vi "Experiment 18.vi"() -> ()   [LabVIEW 2026]
doc: "Experiment 18\nThis experiment is like Experiment 12 but contains only 8 parallel loops (instead of 10 as in Exp 12)."
uses:
  <vilib>/AdvancedString/1D String Array to Delimited String (string).vi
  <vilib>/Analysis/baseanly.llb/Mean (DBL).vi
  <vilib>/Analysis/NI_AALBase.lvlib
panel:
  out "No. Of Iterations As Block Of Text (easy to copy into Excel)":string
  out "No. Of Iterations Executed - Loop 8":i32
  out "Output - Loop 8":dbl[](array[numeric]) format="%.3f"
  out "No. Of Iterations Executed - Loop 7":i32
  out "Output - Loop 7":dbl[](array[numeric]) format="%.3f"
  out "No. Of Iterations Executed - Loop 6":i32
  out "Output - Loop 6":dbl[](array[numeric]) format="%.3f"
  out "No. Of Iterations Executed - Loop 5":i32
  out "Output - Loop 5":dbl[](array[numeric]) format="%.3f"
  out "No. Of Iterations Executed - Loop 4":i32
  out "Output - Loop 4":dbl[](array[numeric]) format="%.3f"
  out "No. Of Iterations Executed - Loop 3":i32
  out "Output - Loop 3":dbl[](array[numeric]) format="%.3f"
  out "Avg. No. Of Iterations Executed - All Loops":dbl format="%.1f"
  out "No. Of Iterations Executed - Loop 2":i32
  out "Output - Loop 2":dbl[](array[numeric]) format="%.3f"
  out "No. Of Iterations Executed - Loop 1":i32
  out "Output - Loop 1":dbl[](array[numeric]) format="%.3f"
  out "Stop VI?":bool
  # "Experiment 18"
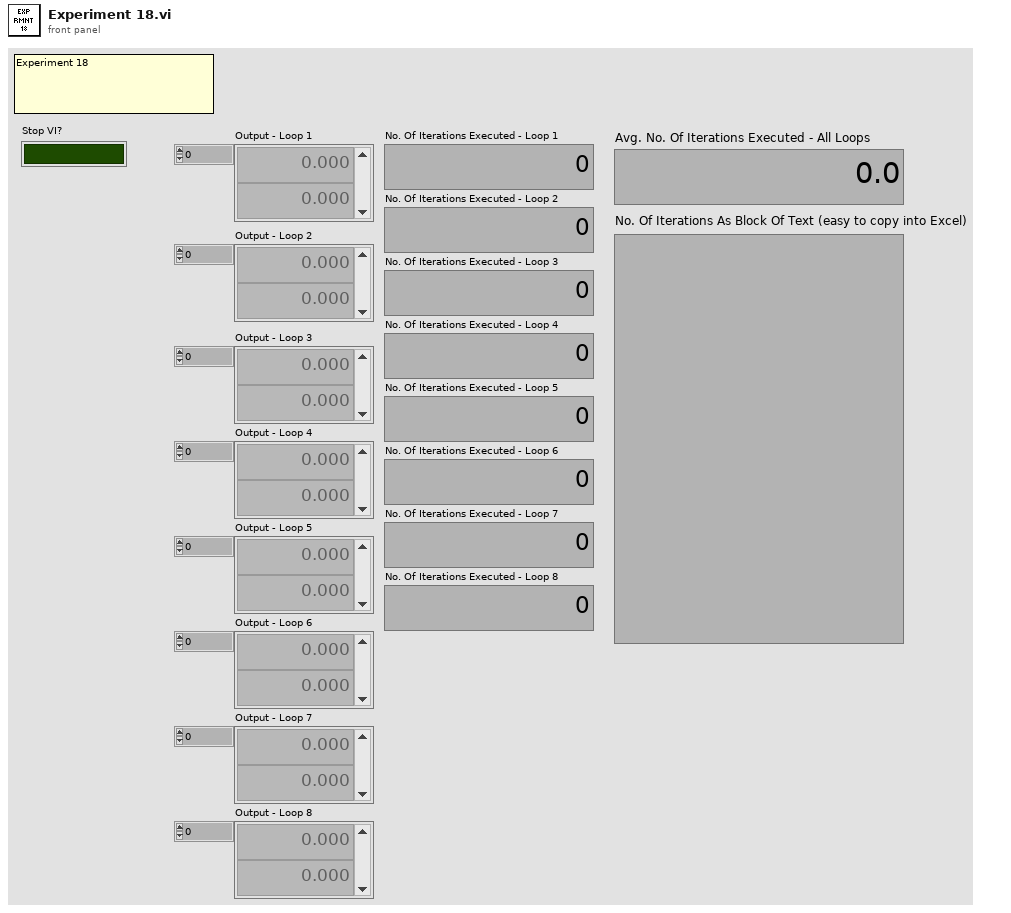
[diagram p1: front panel]
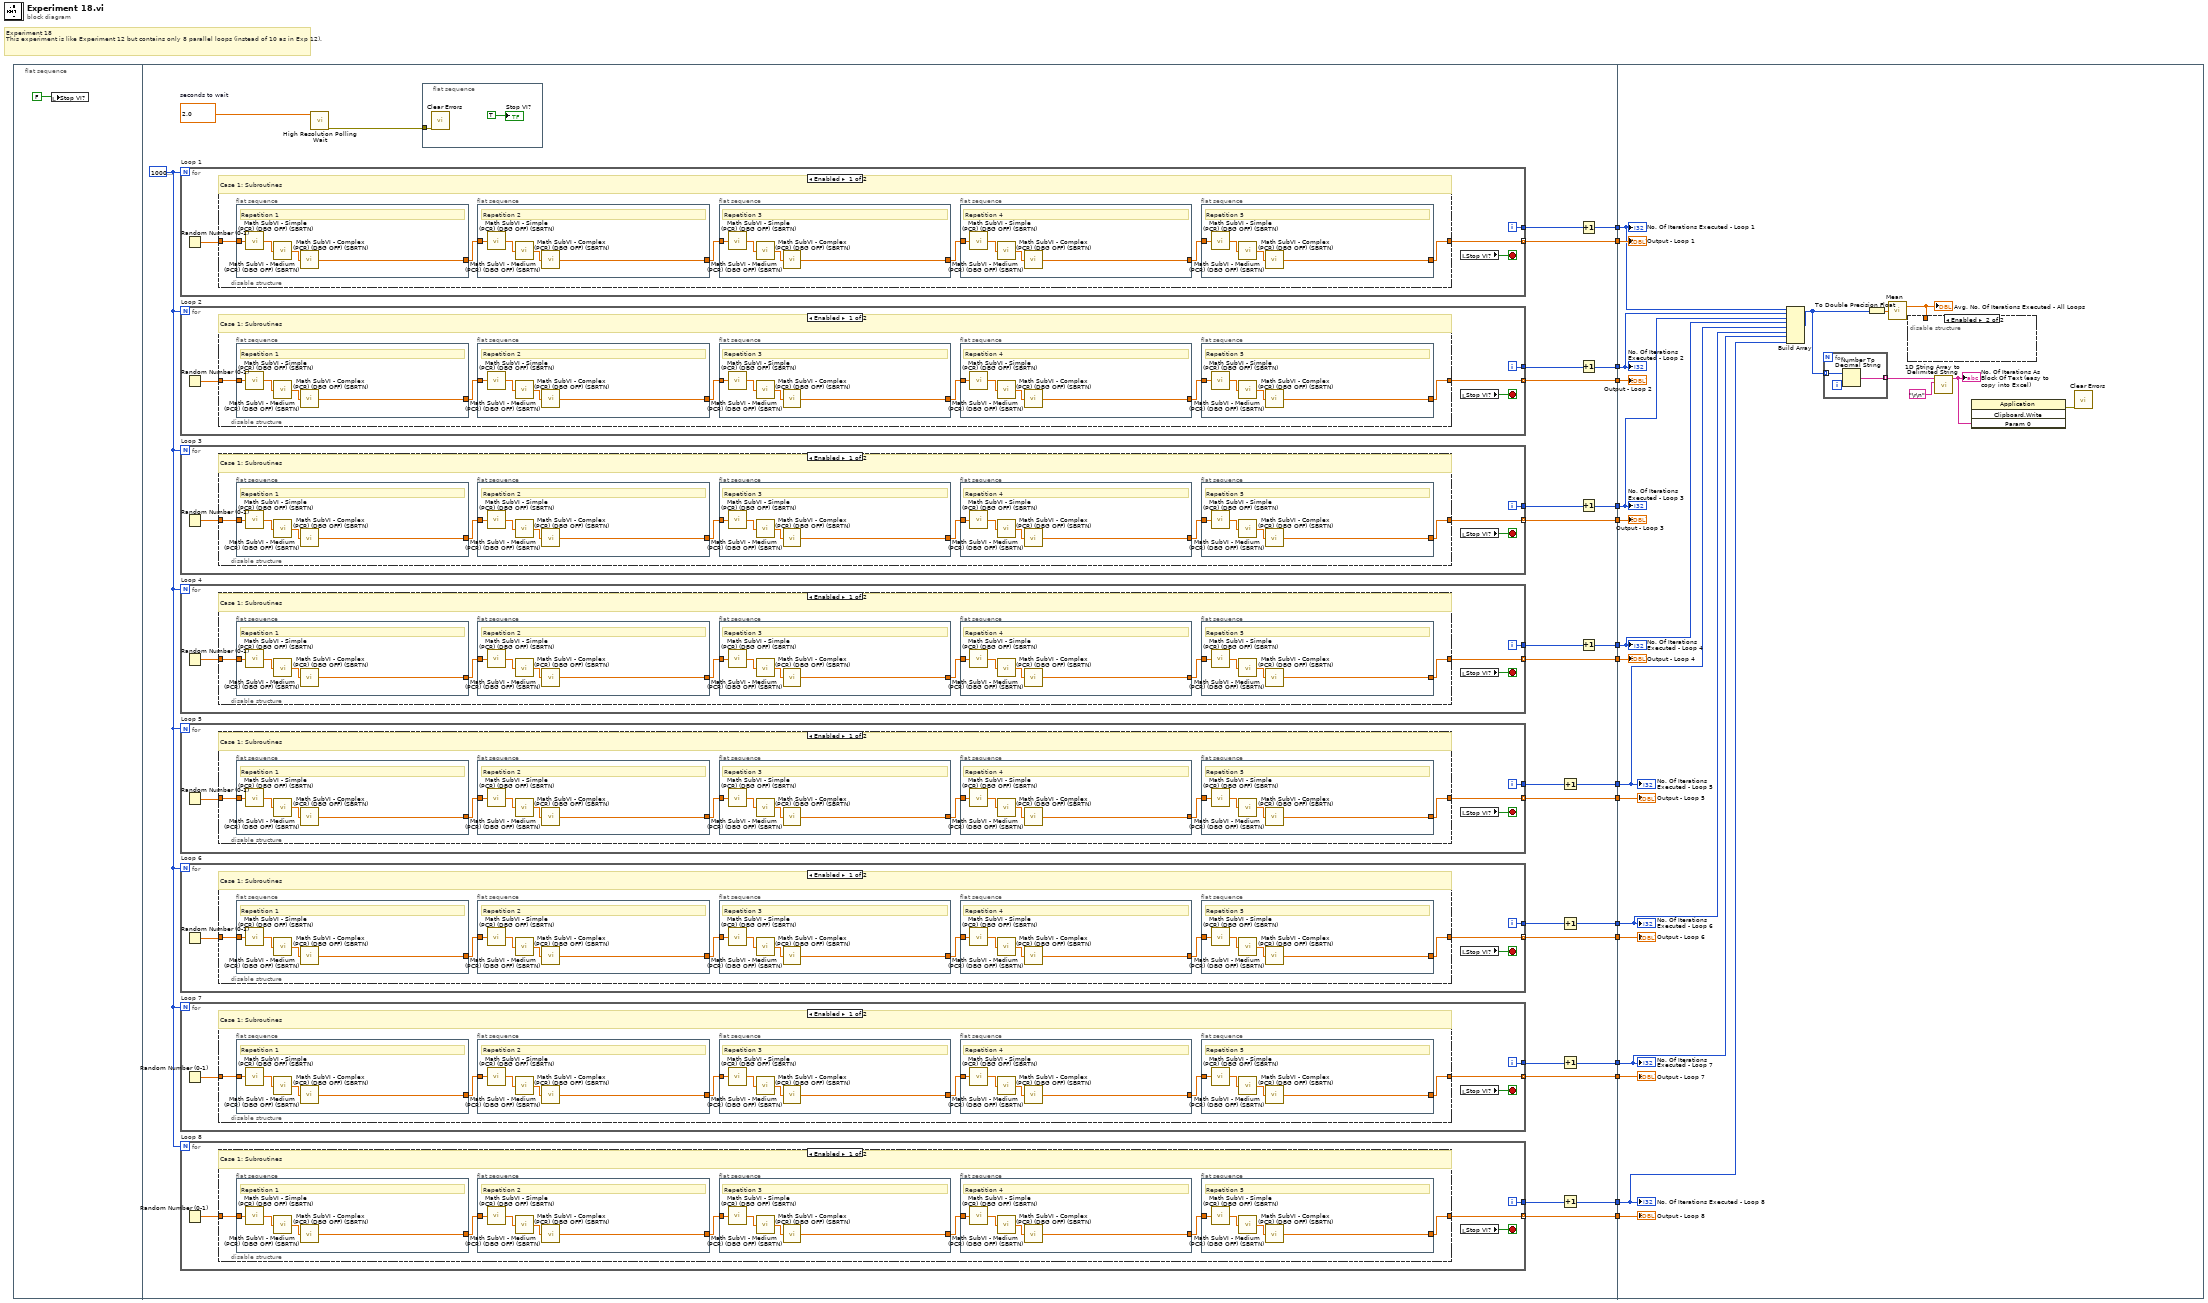
[diagram p0: block diagram]
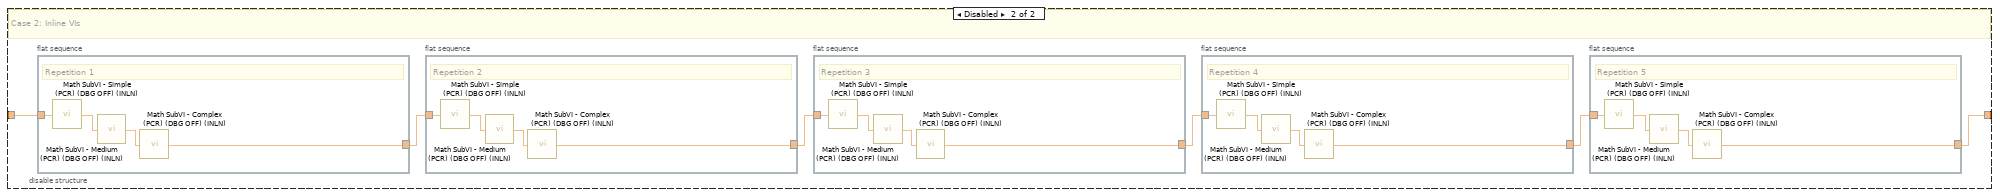
[diagram p2: hidden frame]
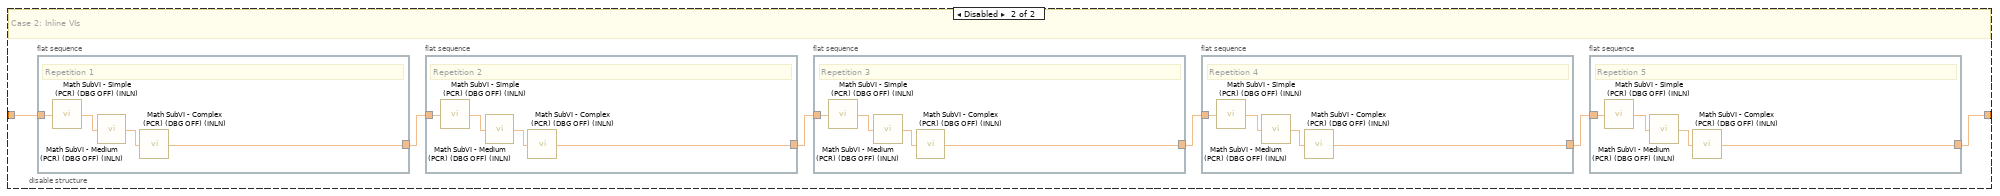
[diagram p3: hidden frame]
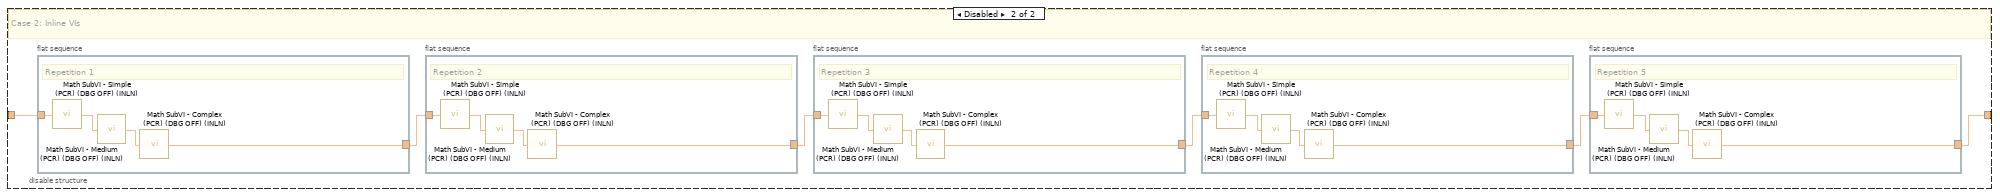
[diagram p4: hidden frame]
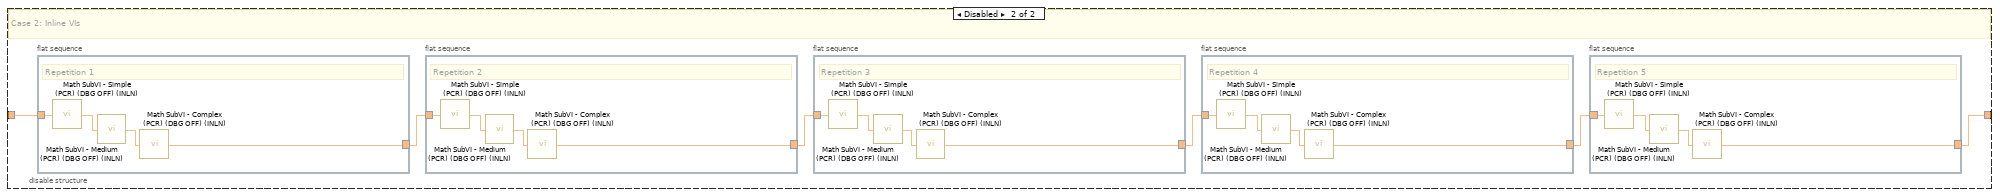
[diagram p5: hidden frame]
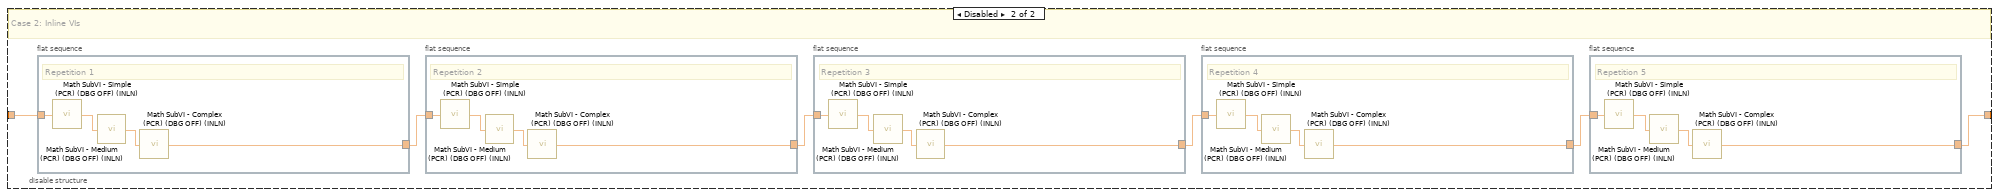
[diagram p6: hidden frame]
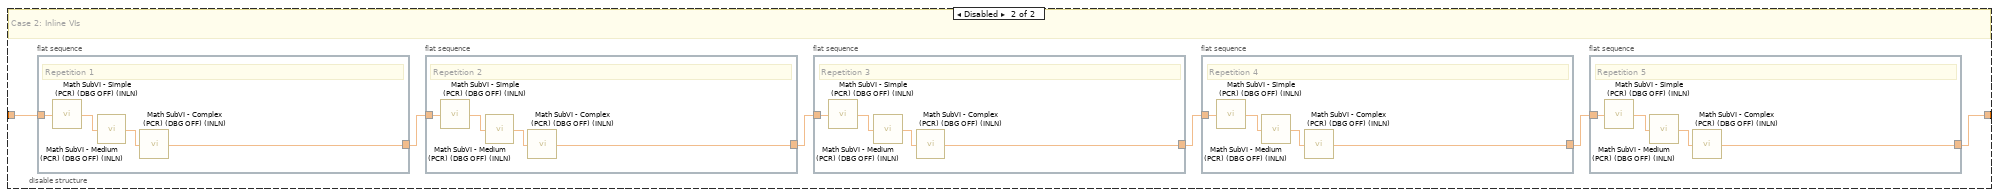
[diagram p7: hidden frame]
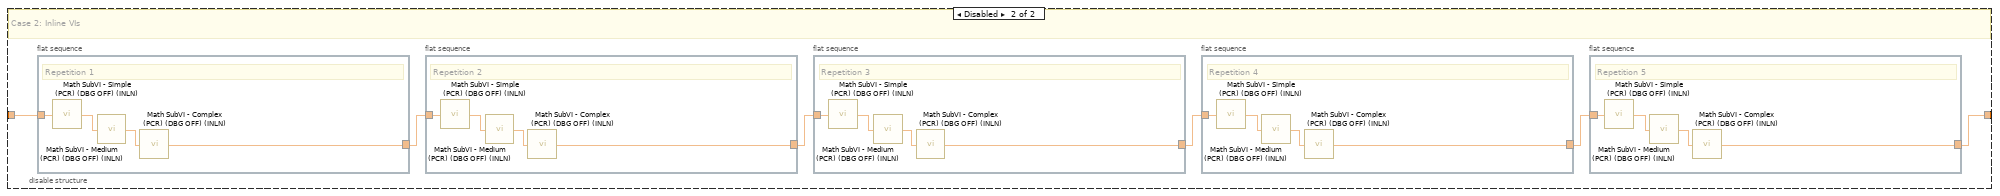
[diagram p8: hidden frame]
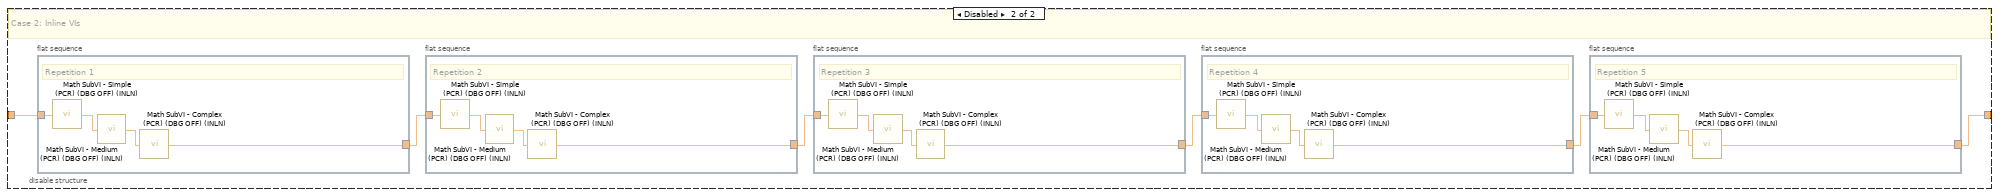
[diagram p9: hidden frame]
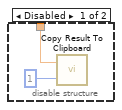
[diagram p10: hidden frame]
diagram:
  # "Experiment 18\nThis experiment is like Experiment 12 but contains only 8 parallel loops (instead of 10 as in Exp 12)."
  n1 = flat-sequence {
    tunnel: [w42] -> w16
    tunnel: [w40] -> w15
    tunnel: [w39] -> w14
    tunnel: [w32] -> w13
    tunnel: [w38] -> w12
    tunnel: [w30] -> w11
    tunnel: [w28] -> w10
    tunnel: [w37] -> w9
    tunnel: [w26] -> w8
    tunnel: [w36] -> w7
    tunnel: [w24] -> w6
    tunnel: [w33] -> w5
    tunnel: [w22] -> w4
    tunnel: [w34] -> w3
    tunnel: [w19] -> w2
    tunnel: [w35] -> w1
    tunnel: w16 -> [w517]
    tunnel: w15 -> [w515]
    tunnel: w14 -> [w514]
    tunnel: w13 -> [w516]
    tunnel: w12 -> [w510]
    tunnel: w11 -> [w512]
    tunnel: w10 -> [w511]
    tunnel: w9 -> [w509]
    tunnel: w8 -> [w507]
    tunnel: w7 -> [w503]
    tunnel: w6 -> [w506]
    tunnel: w5 -> [w502]
    tunnel: w4 -> [w505]
    tunnel: w3 -> [w501]
    tunnel: w2 -> [w504]
    tunnel: w1 -> [w500]
    frame #0 {
      n2 = local write "Stop VI?"(FALSE) -> ()
    }
    frame #1 {
      w18 = 10000000
      w44 = 2.0  # seconds to wait
      n3 = for "Loop 1" {
        N: w18 -> [_]
        tunnel: [w440] -> w42 mode=indexing
        tunnel: [w441] -> w41
        i -> [w441]
        stop <- w442 stop-if-true
        n4 = Random Number (0-1)() -> (number: 0 to 1=w439:dbl)
        n5 = disable-structure shown="Enabled" {
          disable-tunnel: w439 -> [w448 w474]
          disable-tunnel: [w447 w469] -> w440
          frame Enabled {
            # "Case 1: Subroutines"
            n6 = flat-sequence {
              tunnel: w448 -> [w468]
              tunnel: [w465] -> w443
              frame #0 {
                # "Repetition 1"
                n7 = call "Math SubVI - Simple (PCR) (DBG OFF) (SBRTN).vi"("Input"=w468) -> ("Output"=w466:dbl)
                n8 = call "Math SubVI - Medium (PCR) (DBG OFF) (SBRTN).vi"("Input"=w466) -> ("Output"=w467:dbl)
                n9 = call "Math SubVI - Complex (PCR) (DBG OFF) (SBRTN).vi"("Input"=w467) -> ("Output"=w465:dbl)
              }
            }
            n10 = flat-sequence {
              tunnel: w443 -> [w464]
              tunnel: [w461] -> w446
              frame #0 {
                # "Repetition 2"
                n11 = call "Math SubVI - Simple (PCR) (DBG OFF) (SBRTN).vi"("Input"=w464) -> ("Output"=w462:dbl)
                n12 = call "Math SubVI - Medium (PCR) (DBG OFF) (SBRTN).vi"("Input"=w462) -> ("Output"=w463:dbl)
                n13 = call "Math SubVI - Complex (PCR) (DBG OFF) (SBRTN).vi"("Input"=w463) -> ("Output"=w461:dbl)
              }
            }
            n14 = flat-sequence {
              tunnel: w446 -> [w460]
              tunnel: [w457] -> w445
              frame #0 {
                # "Repetition 3"
                n15 = call "Math SubVI - Simple (PCR) (DBG OFF) (SBRTN).vi"("Input"=w460) -> ("Output"=w458:dbl)
                n16 = call "Math SubVI - Medium (PCR) (DBG OFF) (SBRTN).vi"("Input"=w458) -> ("Output"=w459:dbl)
                n17 = call "Math SubVI - Complex (PCR) (DBG OFF) (SBRTN).vi"("Input"=w459) -> ("Output"=w457:dbl)
              }
            }
            n18 = flat-sequence {
              tunnel: w445 -> [w456]
              tunnel: [w453] -> w444
              frame #0 {
                # "Repetition 4"
                n19 = call "Math SubVI - Simple (PCR) (DBG OFF) (SBRTN).vi"("Input"=w456) -> ("Output"=w454:dbl)
                n20 = call "Math SubVI - Medium (PCR) (DBG OFF) (SBRTN).vi"("Input"=w454) -> ("Output"=w455:dbl)
                n21 = call "Math SubVI - Complex (PCR) (DBG OFF) (SBRTN).vi"("Input"=w455) -> ("Output"=w453:dbl)
              }
            }
            n22 = flat-sequence {
              tunnel: w444 -> [w452]
              tunnel: [w449] -> w447
              frame #0 {
                # "Repetition 5"
                n23 = call "Math SubVI - Simple (PCR) (DBG OFF) (SBRTN).vi"("Input"=w452) -> ("Output"=w450:dbl)
                n24 = call "Math SubVI - Medium (PCR) (DBG OFF) (SBRTN).vi"("Input"=w450) -> ("Output"=w451:dbl)
                n25 = call "Math SubVI - Complex (PCR) (DBG OFF) (SBRTN).vi"("Input"=w451) -> ("Output"=w449:dbl)
              }
            }
          }
          frame Disabled {
            # "Case 2: Inline VIs"
            n26 = flat-sequence {
              tunnel: w474 -> [w494]
              tunnel: [w491] -> w473
              frame #0 {
                # "Repetition 1"
                n27 = call "Math SubVI - Simple (PCR) (DBG OFF) (INLN).vi"("Input"=w494) -> ("Output"=w492:dbl)
                n28 = call "Math SubVI - Medium (PCR) (DBG OFF) (INLN).vi"("Input"=w492) -> ("Output"=w493:dbl)
                n29 = call "Math SubVI - Complex (PCR) (DBG OFF) (INLN).vi"("Input"=w493) -> ("Output"=w491:dbl)
              }
            }
            n30 = flat-sequence {
              tunnel: w473 -> [w490]
              tunnel: [w487] -> w472
              frame #0 {
                # "Repetition 2"
                n31 = call "Math SubVI - Simple (PCR) (DBG OFF) (INLN).vi"("Input"=w490) -> ("Output"=w488:dbl)
                n32 = call "Math SubVI - Medium (PCR) (DBG OFF) (INLN).vi"("Input"=w488) -> ("Output"=w489:dbl)
                n33 = call "Math SubVI - Complex (PCR) (DBG OFF) (INLN).vi"("Input"=w489) -> ("Output"=w487:dbl)
              }
            }
            n34 = flat-sequence {
              tunnel: w472 -> [w486]
              tunnel: [w483] -> w471
              frame #0 {
                # "Repetition 3"
                n35 = call "Math SubVI - Simple (PCR) (DBG OFF) (INLN).vi"("Input"=w486) -> ("Output"=w484:dbl)
                n36 = call "Math SubVI - Medium (PCR) (DBG OFF) (INLN).vi"("Input"=w484) -> ("Output"=w485:dbl)
                n37 = call "Math SubVI - Complex (PCR) (DBG OFF) (INLN).vi"("Input"=w485) -> ("Output"=w483:dbl)
              }
            }
            n38 = flat-sequence {
              tunnel: w471 -> [w482]
              tunnel: [w479] -> w470
              frame #0 {
                # "Repetition 4"
                n39 = call "Math SubVI - Simple (PCR) (DBG OFF) (INLN).vi"("Input"=w482) -> ("Output"=w480:dbl)
                n40 = call "Math SubVI - Medium (PCR) (DBG OFF) (INLN).vi"("Input"=w480) -> ("Output"=w481:dbl)
                n41 = call "Math SubVI - Complex (PCR) (DBG OFF) (INLN).vi"("Input"=w481) -> ("Output"=w479:dbl)
              }
            }
            n42 = flat-sequence {
              tunnel: w470 -> [w478]
              tunnel: [w475] -> w469
              frame #0 {
                # "Repetition 5"
                n43 = call "Math SubVI - Simple (PCR) (DBG OFF) (INLN).vi"("Input"=w478) -> ("Output"=w476:dbl)
                n44 = call "Math SubVI - Medium (PCR) (DBG OFF) (INLN).vi"("Input"=w476) -> ("Output"=w477:dbl)
                n45 = call "Math SubVI - Complex (PCR) (DBG OFF) (INLN).vi"("Input"=w477) -> ("Output"=w475:dbl)
              }
            }
          }
        }
        n46 = local read "Stop VI?"() -> (w442:bool)
      }
      n47 = for "Loop 2" {
        N: w18 -> [_]
        tunnel: [w384] -> w32 mode=indexing
        tunnel: [w385] -> w31
        i -> [w385]
        stop <- w386 stop-if-true
        n48 = Random Number (0-1)() -> (number: 0 to 1=w383:dbl)
        n49 = disable-structure shown="Enabled" {
          disable-tunnel: w383 -> [w392 w418]
          disable-tunnel: [w391 w413] -> w384
          frame Enabled {
            # "Case 1: Subroutines"
            n50 = flat-sequence {
              tunnel: w392 -> [w412]
              tunnel: [w409] -> w387
              frame #0 {
                # "Repetition 1"
                n51 = call "Math SubVI - Simple (PCR) (DBG OFF) (SBRTN).vi"("Input"=w412) -> ("Output"=w410:dbl)
                n52 = call "Math SubVI - Medium (PCR) (DBG OFF) (SBRTN).vi"("Input"=w410) -> ("Output"=w411:dbl)
                n53 = call "Math SubVI - Complex (PCR) (DBG OFF) (SBRTN).vi"("Input"=w411) -> ("Output"=w409:dbl)
              }
            }
            n54 = flat-sequence {
              tunnel: w387 -> [w408]
              tunnel: [w405] -> w390
              frame #0 {
                # "Repetition 2"
                n55 = call "Math SubVI - Simple (PCR) (DBG OFF) (SBRTN).vi"("Input"=w408) -> ("Output"=w406:dbl)
                n56 = call "Math SubVI - Medium (PCR) (DBG OFF) (SBRTN).vi"("Input"=w406) -> ("Output"=w407:dbl)
                n57 = call "Math SubVI - Complex (PCR) (DBG OFF) (SBRTN).vi"("Input"=w407) -> ("Output"=w405:dbl)
              }
            }
            n58 = flat-sequence {
              tunnel: w390 -> [w404]
              tunnel: [w401] -> w389
              frame #0 {
                # "Repetition 3"
                n59 = call "Math SubVI - Simple (PCR) (DBG OFF) (SBRTN).vi"("Input"=w404) -> ("Output"=w402:dbl)
                n60 = call "Math SubVI - Medium (PCR) (DBG OFF) (SBRTN).vi"("Input"=w402) -> ("Output"=w403:dbl)
                n61 = call "Math SubVI - Complex (PCR) (DBG OFF) (SBRTN).vi"("Input"=w403) -> ("Output"=w401:dbl)
              }
            }
            n62 = flat-sequence {
              tunnel: w389 -> [w400]
              tunnel: [w397] -> w388
              frame #0 {
                # "Repetition 4"
                n63 = call "Math SubVI - Simple (PCR) (DBG OFF) (SBRTN).vi"("Input"=w400) -> ("Output"=w398:dbl)
                n64 = call "Math SubVI - Medium (PCR) (DBG OFF) (SBRTN).vi"("Input"=w398) -> ("Output"=w399:dbl)
                n65 = call "Math SubVI - Complex (PCR) (DBG OFF) (SBRTN).vi"("Input"=w399) -> ("Output"=w397:dbl)
              }
            }
            n66 = flat-sequence {
              tunnel: w388 -> [w396]
              tunnel: [w393] -> w391
              frame #0 {
                # "Repetition 5"
                n67 = call "Math SubVI - Simple (PCR) (DBG OFF) (SBRTN).vi"("Input"=w396) -> ("Output"=w394:dbl)
                n68 = call "Math SubVI - Medium (PCR) (DBG OFF) (SBRTN).vi"("Input"=w394) -> ("Output"=w395:dbl)
                n69 = call "Math SubVI - Complex (PCR) (DBG OFF) (SBRTN).vi"("Input"=w395) -> ("Output"=w393:dbl)
              }
            }
          }
          frame Disabled {
            # "Case 2: Inline VIs"
            n70 = flat-sequence {
              tunnel: w418 -> [w438]
              tunnel: [w435] -> w417
              frame #0 {
                # "Repetition 1"
                n71 = call "Math SubVI - Simple (PCR) (DBG OFF) (INLN).vi"("Input"=w438) -> ("Output"=w436:dbl)
                n72 = call "Math SubVI - Medium (PCR) (DBG OFF) (INLN).vi"("Input"=w436) -> ("Output"=w437:dbl)
                n73 = call "Math SubVI - Complex (PCR) (DBG OFF) (INLN).vi"("Input"=w437) -> ("Output"=w435:dbl)
              }
            }
            n74 = flat-sequence {
              tunnel: w417 -> [w434]
              tunnel: [w431] -> w416
              frame #0 {
                # "Repetition 2"
                n75 = call "Math SubVI - Simple (PCR) (DBG OFF) (INLN).vi"("Input"=w434) -> ("Output"=w432:dbl)
                n76 = call "Math SubVI - Medium (PCR) (DBG OFF) (INLN).vi"("Input"=w432) -> ("Output"=w433:dbl)
                n77 = call "Math SubVI - Complex (PCR) (DBG OFF) (INLN).vi"("Input"=w433) -> ("Output"=w431:dbl)
              }
            }
            n78 = flat-sequence {
              tunnel: w416 -> [w430]
              tunnel: [w427] -> w415
              frame #0 {
                # "Repetition 3"
                n79 = call "Math SubVI - Simple (PCR) (DBG OFF) (INLN).vi"("Input"=w430) -> ("Output"=w428:dbl)
                n80 = call "Math SubVI - Medium (PCR) (DBG OFF) (INLN).vi"("Input"=w428) -> ("Output"=w429:dbl)
                n81 = call "Math SubVI - Complex (PCR) (DBG OFF) (INLN).vi"("Input"=w429) -> ("Output"=w427:dbl)
              }
            }
            n82 = flat-sequence {
              tunnel: w415 -> [w426]
              tunnel: [w423] -> w414
              frame #0 {
                # "Repetition 4"
                n83 = call "Math SubVI - Simple (PCR) (DBG OFF) (INLN).vi"("Input"=w426) -> ("Output"=w424:dbl)
                n84 = call "Math SubVI - Medium (PCR) (DBG OFF) (INLN).vi"("Input"=w424) -> ("Output"=w425:dbl)
                n85 = call "Math SubVI - Complex (PCR) (DBG OFF) (INLN).vi"("Input"=w425) -> ("Output"=w423:dbl)
              }
            }
            n86 = flat-sequence {
              tunnel: w414 -> [w422]
              tunnel: [w419] -> w413
              frame #0 {
                # "Repetition 5"
                n87 = call "Math SubVI - Simple (PCR) (DBG OFF) (INLN).vi"("Input"=w422) -> ("Output"=w420:dbl)
                n88 = call "Math SubVI - Medium (PCR) (DBG OFF) (INLN).vi"("Input"=w420) -> ("Output"=w421:dbl)
                n89 = call "Math SubVI - Complex (PCR) (DBG OFF) (INLN).vi"("Input"=w421) -> ("Output"=w419:dbl)
              }
            }
          }
        }
        n90 = local read "Stop VI?"() -> (w386:bool)
      }
      n91 = for "Loop 3" {
        N: w18 -> [_]
        tunnel: [w328] -> w30 mode=indexing
        tunnel: [w329] -> w29
        i -> [w329]
        stop <- w330 stop-if-true
        n92 = Random Number (0-1)() -> (number: 0 to 1=w327:dbl)
        n93 = disable-structure shown="Enabled" {
          disable-tunnel: w327 -> [w336 w362]
          disable-tunnel: [w335 w357] -> w328
          frame Enabled {
            # "Case 1: Subroutines"
            n94 = flat-sequence {
              tunnel: w336 -> [w356]
              tunnel: [w353] -> w331
              frame #0 {
                # "Repetition 1"
                n95 = call "Math SubVI - Simple (PCR) (DBG OFF) (SBRTN).vi"("Input"=w356) -> ("Output"=w354:dbl)
                n96 = call "Math SubVI - Medium (PCR) (DBG OFF) (SBRTN).vi"("Input"=w354) -> ("Output"=w355:dbl)
                n97 = call "Math SubVI - Complex (PCR) (DBG OFF) (SBRTN).vi"("Input"=w355) -> ("Output"=w353:dbl)
              }
            }
            n98 = flat-sequence {
              tunnel: w331 -> [w352]
              tunnel: [w349] -> w334
              frame #0 {
                # "Repetition 2"
                n99 = call "Math SubVI - Simple (PCR) (DBG OFF) (SBRTN).vi"("Input"=w352) -> ("Output"=w350:dbl)
                n100 = call "Math SubVI - Medium (PCR) (DBG OFF) (SBRTN).vi"("Input"=w350) -> ("Output"=w351:dbl)
                n101 = call "Math SubVI - Complex (PCR) (DBG OFF) (SBRTN).vi"("Input"=w351) -> ("Output"=w349:dbl)
              }
            }
            n102 = flat-sequence {
              tunnel: w334 -> [w348]
              tunnel: [w345] -> w333
              frame #0 {
                # "Repetition 3"
                n103 = call "Math SubVI - Simple (PCR) (DBG OFF) (SBRTN).vi"("Input"=w348) -> ("Output"=w346:dbl)
                n104 = call "Math SubVI - Medium (PCR) (DBG OFF) (SBRTN).vi"("Input"=w346) -> ("Output"=w347:dbl)
                n105 = call "Math SubVI - Complex (PCR) (DBG OFF) (SBRTN).vi"("Input"=w347) -> ("Output"=w345:dbl)
              }
            }
            n106 = flat-sequence {
              tunnel: w333 -> [w344]
              tunnel: [w341] -> w332
              frame #0 {
                # "Repetition 4"
                n107 = call "Math SubVI - Simple (PCR) (DBG OFF) (SBRTN).vi"("Input"=w344) -> ("Output"=w342:dbl)
                n108 = call "Math SubVI - Medium (PCR) (DBG OFF) (SBRTN).vi"("Input"=w342) -> ("Output"=w343:dbl)
                n109 = call "Math SubVI - Complex (PCR) (DBG OFF) (SBRTN).vi"("Input"=w343) -> ("Output"=w341:dbl)
              }
            }
            n110 = flat-sequence {
              tunnel: w332 -> [w340]
              tunnel: [w337] -> w335
              frame #0 {
                # "Repetition 5"
                n111 = call "Math SubVI - Simple (PCR) (DBG OFF) (SBRTN).vi"("Input"=w340) -> ("Output"=w338:dbl)
                n112 = call "Math SubVI - Medium (PCR) (DBG OFF) (SBRTN).vi"("Input"=w338) -> ("Output"=w339:dbl)
                n113 = call "Math SubVI - Complex (PCR) (DBG OFF) (SBRTN).vi"("Input"=w339) -> ("Output"=w337:dbl)
              }
            }
          }
          frame Disabled {
            # "Case 2: Inline VIs"
            n114 = flat-sequence {
              tunnel: w362 -> [w382]
              tunnel: [w379] -> w361
              frame #0 {
                # "Repetition 1"
                n115 = call "Math SubVI - Simple (PCR) (DBG OFF) (INLN).vi"("Input"=w382) -> ("Output"=w380:dbl)
                n116 = call "Math SubVI - Medium (PCR) (DBG OFF) (INLN).vi"("Input"=w380) -> ("Output"=w381:dbl)
                n117 = call "Math SubVI - Complex (PCR) (DBG OFF) (INLN).vi"("Input"=w381) -> ("Output"=w379:dbl)
              }
            }
            n118 = flat-sequence {
              tunnel: w361 -> [w378]
              tunnel: [w375] -> w360
              frame #0 {
                # "Repetition 2"
                n119 = call "Math SubVI - Simple (PCR) (DBG OFF) (INLN).vi"("Input"=w378) -> ("Output"=w376:dbl)
                n120 = call "Math SubVI - Medium (PCR) (DBG OFF) (INLN).vi"("Input"=w376) -> ("Output"=w377:dbl)
                n121 = call "Math SubVI - Complex (PCR) (DBG OFF) (INLN).vi"("Input"=w377) -> ("Output"=w375:dbl)
              }
            }
            n122 = flat-sequence {
              tunnel: w360 -> [w374]
              tunnel: [w371] -> w359
              frame #0 {
                # "Repetition 3"
                n123 = call "Math SubVI - Simple (PCR) (DBG OFF) (INLN).vi"("Input"=w374) -> ("Output"=w372:dbl)
                n124 = call "Math SubVI - Medium (PCR) (DBG OFF) (INLN).vi"("Input"=w372) -> ("Output"=w373:dbl)
                n125 = call "Math SubVI - Complex (PCR) (DBG OFF) (INLN).vi"("Input"=w373) -> ("Output"=w371:dbl)
              }
            }
            n126 = flat-sequence {
              tunnel: w359 -> [w370]
              tunnel: [w367] -> w358
              frame #0 {
                # "Repetition 4"
                n127 = call "Math SubVI - Simple (PCR) (DBG OFF) (INLN).vi"("Input"=w370) -> ("Output"=w368:dbl)
                n128 = call "Math SubVI - Medium (PCR) (DBG OFF) (INLN).vi"("Input"=w368) -> ("Output"=w369:dbl)
                n129 = call "Math SubVI - Complex (PCR) (DBG OFF) (INLN).vi"("Input"=w369) -> ("Output"=w367:dbl)
              }
            }
            n130 = flat-sequence {
              tunnel: w358 -> [w366]
              tunnel: [w363] -> w357
              frame #0 {
                # "Repetition 5"
                n131 = call "Math SubVI - Simple (PCR) (DBG OFF) (INLN).vi"("Input"=w366) -> ("Output"=w364:dbl)
                n132 = call "Math SubVI - Medium (PCR) (DBG OFF) (INLN).vi"("Input"=w364) -> ("Output"=w365:dbl)
                n133 = call "Math SubVI - Complex (PCR) (DBG OFF) (INLN).vi"("Input"=w365) -> ("Output"=w363:dbl)
              }
            }
          }
        }
        n134 = local read "Stop VI?"() -> (w330:bool)
      }
      n135 = for "Loop 4" {
        N: w18 -> [_]
        tunnel: [w272] -> w28 mode=indexing
        tunnel: [w273] -> w27
        i -> [w273]
        stop <- w274 stop-if-true
        n136 = Random Number (0-1)() -> (number: 0 to 1=w271:dbl)
        n137 = disable-structure shown="Enabled" {
          disable-tunnel: w271 -> [w280 w306]
          disable-tunnel: [w279 w301] -> w272
          frame Enabled {
            # "Case 1: Subroutines"
            n138 = flat-sequence {
              tunnel: w280 -> [w300]
              tunnel: [w297] -> w275
              frame #0 {
                # "Repetition 1"
                n139 = call "Math SubVI - Simple (PCR) (DBG OFF) (SBRTN).vi"("Input"=w300) -> ("Output"=w298:dbl)
                n140 = call "Math SubVI - Medium (PCR) (DBG OFF) (SBRTN).vi"("Input"=w298) -> ("Output"=w299:dbl)
                n141 = call "Math SubVI - Complex (PCR) (DBG OFF) (SBRTN).vi"("Input"=w299) -> ("Output"=w297:dbl)
              }
            }
            n142 = flat-sequence {
              tunnel: w275 -> [w296]
              tunnel: [w293] -> w278
              frame #0 {
                # "Repetition 2"
                n143 = call "Math SubVI - Simple (PCR) (DBG OFF) (SBRTN).vi"("Input"=w296) -> ("Output"=w294:dbl)
                n144 = call "Math SubVI - Medium (PCR) (DBG OFF) (SBRTN).vi"("Input"=w294) -> ("Output"=w295:dbl)
                n145 = call "Math SubVI - Complex (PCR) (DBG OFF) (SBRTN).vi"("Input"=w295) -> ("Output"=w293:dbl)
              }
            }
            n146 = flat-sequence {
              tunnel: w278 -> [w292]
              tunnel: [w289] -> w277
              frame #0 {
                # "Repetition 3"
                n147 = call "Math SubVI - Simple (PCR) (DBG OFF) (SBRTN).vi"("Input"=w292) -> ("Output"=w290:dbl)
                n148 = call "Math SubVI - Medium (PCR) (DBG OFF) (SBRTN).vi"("Input"=w290) -> ("Output"=w291:dbl)
                n149 = call "Math SubVI - Complex (PCR) (DBG OFF) (SBRTN).vi"("Input"=w291) -> ("Output"=w289:dbl)
              }
            }
            n150 = flat-sequence {
              tunnel: w277 -> [w288]
              tunnel: [w285] -> w276
              frame #0 {
                # "Repetition 4"
                n151 = call "Math SubVI - Simple (PCR) (DBG OFF) (SBRTN).vi"("Input"=w288) -> ("Output"=w286:dbl)
                n152 = call "Math SubVI - Medium (PCR) (DBG OFF) (SBRTN).vi"("Input"=w286) -> ("Output"=w287:dbl)
                n153 = call "Math SubVI - Complex (PCR) (DBG OFF) (SBRTN).vi"("Input"=w287) -> ("Output"=w285:dbl)
              }
            }
            n154 = flat-sequence {
              tunnel: w276 -> [w284]
              tunnel: [w281] -> w279
              frame #0 {
                # "Repetition 5"
                n155 = call "Math SubVI - Simple (PCR) (DBG OFF) (SBRTN).vi"("Input"=w284) -> ("Output"=w282:dbl)
                n156 = call "Math SubVI - Medium (PCR) (DBG OFF) (SBRTN).vi"("Input"=w282) -> ("Output"=w283:dbl)
                n157 = call "Math SubVI - Complex (PCR) (DBG OFF) (SBRTN).vi"("Input"=w283) -> ("Output"=w281:dbl)
              }
            }
          }
          frame Disabled {
            # "Case 2: Inline VIs"
            n158 = flat-sequence {
              tunnel: w306 -> [w326]
              tunnel: [w323] -> w305
              frame #0 {
                # "Repetition 1"
                n159 = call "Math SubVI - Simple (PCR) (DBG OFF) (INLN).vi"("Input"=w326) -> ("Output"=w324:dbl)
                n160 = call "Math SubVI - Medium (PCR) (DBG OFF) (INLN).vi"("Input"=w324) -> ("Output"=w325:dbl)
                n161 = call "Math SubVI - Complex (PCR) (DBG OFF) (INLN).vi"("Input"=w325) -> ("Output"=w323:dbl)
              }
            }
            n162 = flat-sequence {
              tunnel: w305 -> [w322]
              tunnel: [w319] -> w304
              frame #0 {
                # "Repetition 2"
                n163 = call "Math SubVI - Simple (PCR) (DBG OFF) (INLN).vi"("Input"=w322) -> ("Output"=w320:dbl)
                n164 = call "Math SubVI - Medium (PCR) (DBG OFF) (INLN).vi"("Input"=w320) -> ("Output"=w321:dbl)
                n165 = call "Math SubVI - Complex (PCR) (DBG OFF) (INLN).vi"("Input"=w321) -> ("Output"=w319:dbl)
              }
            }
            n166 = flat-sequence {
              tunnel: w304 -> [w318]
              tunnel: [w315] -> w303
              frame #0 {
                # "Repetition 3"
                n167 = call "Math SubVI - Simple (PCR) (DBG OFF) (INLN).vi"("Input"=w318) -> ("Output"=w316:dbl)
                n168 = call "Math SubVI - Medium (PCR) (DBG OFF) (INLN).vi"("Input"=w316) -> ("Output"=w317:dbl)
                n169 = call "Math SubVI - Complex (PCR) (DBG OFF) (INLN).vi"("Input"=w317) -> ("Output"=w315:dbl)
              }
            }
            n170 = flat-sequence {
              tunnel: w303 -> [w314]
              tunnel: [w311] -> w302
              frame #0 {
                # "Repetition 4"
                n171 = call "Math SubVI - Simple (PCR) (DBG OFF) (INLN).vi"("Input"=w314) -> ("Output"=w312:dbl)
                n172 = call "Math SubVI - Medium (PCR) (DBG OFF) (INLN).vi"("Input"=w312) -> ("Output"=w313:dbl)
                n173 = call "Math SubVI - Complex (PCR) (DBG OFF) (INLN).vi"("Input"=w313) -> ("Output"=w311:dbl)
              }
            }
            n174 = flat-sequence {
              tunnel: w302 -> [w310]
              tunnel: [w307] -> w301
              frame #0 {
                # "Repetition 5"
                n175 = call "Math SubVI - Simple (PCR) (DBG OFF) (INLN).vi"("Input"=w310) -> ("Output"=w308:dbl)
                n176 = call "Math SubVI - Medium (PCR) (DBG OFF) (INLN).vi"("Input"=w308) -> ("Output"=w309:dbl)
                n177 = call "Math SubVI - Complex (PCR) (DBG OFF) (INLN).vi"("Input"=w309) -> ("Output"=w307:dbl)
              }
            }
          }
        }
        n178 = local read "Stop VI?"() -> (w274:bool)
      }
      n179 = for "Loop 5" {
        N: w18 -> [_]
        tunnel: [w216] -> w26 mode=indexing
        tunnel: [w217] -> w25
        i -> [w217]
        stop <- w218 stop-if-true
        n180 = Random Number (0-1)() -> (number: 0 to 1=w215:dbl)
        n181 = disable-structure shown="Enabled" {
          disable-tunnel: w215 -> [w224 w250]
          disable-tunnel: [w223 w245] -> w216
          frame Enabled {
            # "Case 1: Subroutines"
            n182 = flat-sequence {
              tunnel: w224 -> [w244]
              tunnel: [w241] -> w219
              frame #0 {
                # "Repetition 1"
                n183 = call "Math SubVI - Simple (PCR) (DBG OFF) (SBRTN).vi"("Input"=w244) -> ("Output"=w242:dbl)
                n184 = call "Math SubVI - Medium (PCR) (DBG OFF) (SBRTN).vi"("Input"=w242) -> ("Output"=w243:dbl)
                n185 = call "Math SubVI - Complex (PCR) (DBG OFF) (SBRTN).vi"("Input"=w243) -> ("Output"=w241:dbl)
              }
            }
            n186 = flat-sequence {
              tunnel: w219 -> [w240]
              tunnel: [w237] -> w222
              frame #0 {
                # "Repetition 2"
                n187 = call "Math SubVI - Simple (PCR) (DBG OFF) (SBRTN).vi"("Input"=w240) -> ("Output"=w238:dbl)
                n188 = call "Math SubVI - Medium (PCR) (DBG OFF) (SBRTN).vi"("Input"=w238) -> ("Output"=w239:dbl)
                n189 = call "Math SubVI - Complex (PCR) (DBG OFF) (SBRTN).vi"("Input"=w239) -> ("Output"=w237:dbl)
              }
            }
            n190 = flat-sequence {
              tunnel: w222 -> [w236]
              tunnel: [w233] -> w221
              frame #0 {
                # "Repetition 3"
                n191 = call "Math SubVI - Simple (PCR) (DBG OFF) (SBRTN).vi"("Input"=w236) -> ("Output"=w234:dbl)
                n192 = call "Math SubVI - Medium (PCR) (DBG OFF) (SBRTN).vi"("Input"=w234) -> ("Output"=w235:dbl)
                n193 = call "Math SubVI - Complex (PCR) (DBG OFF) (SBRTN).vi"("Input"=w235) -> ("Output"=w233:dbl)
              }
            }
            n194 = flat-sequence {
              tunnel: w221 -> [w232]
              tunnel: [w229] -> w220
              frame #0 {
                # "Repetition 4"
                n195 = call "Math SubVI - Simple (PCR) (DBG OFF) (SBRTN).vi"("Input"=w232) -> ("Output"=w230:dbl)
                n196 = call "Math SubVI - Medium (PCR) (DBG OFF) (SBRTN).vi"("Input"=w230) -> ("Output"=w231:dbl)
                n197 = call "Math SubVI - Complex (PCR) (DBG OFF) (SBRTN).vi"("Input"=w231) -> ("Output"=w229:dbl)
              }
            }
            n198 = flat-sequence {
              tunnel: w220 -> [w228]
              tunnel: [w225] -> w223
              frame #0 {
                # "Repetition 5"
                n199 = call "Math SubVI - Simple (PCR) (DBG OFF) (SBRTN).vi"("Input"=w228) -> ("Output"=w226:dbl)
                n200 = call "Math SubVI - Medium (PCR) (DBG OFF) (SBRTN).vi"("Input"=w226) -> ("Output"=w227:dbl)
                n201 = call "Math SubVI - Complex (PCR) (DBG OFF) (SBRTN).vi"("Input"=w227) -> ("Output"=w225:dbl)
              }
            }
          }
          frame Disabled {
            # "Case 2: Inline VIs"
            n202 = flat-sequence {
              tunnel: w250 -> [w270]
              tunnel: [w267] -> w249
              frame #0 {
                # "Repetition 1"
                n203 = call "Math SubVI - Simple (PCR) (DBG OFF) (INLN).vi"("Input"=w270) -> ("Output"=w268:dbl)
                n204 = call "Math SubVI - Medium (PCR) (DBG OFF) (INLN).vi"("Input"=w268) -> ("Output"=w269:dbl)
                n205 = call "Math SubVI - Complex (PCR) (DBG OFF) (INLN).vi"("Input"=w269) -> ("Output"=w267:dbl)
              }
            }
            n206 = flat-sequence {
              tunnel: w249 -> [w266]
              tunnel: [w263] -> w248
              frame #0 {
                # "Repetition 2"
                n207 = call "Math SubVI - Simple (PCR) (DBG OFF) (INLN).vi"("Input"=w266) -> ("Output"=w264:dbl)
                n208 = call "Math SubVI - Medium (PCR) (DBG OFF) (INLN).vi"("Input"=w264) -> ("Output"=w265:dbl)
                n209 = call "Math SubVI - Complex (PCR) (DBG OFF) (INLN).vi"("Input"=w265) -> ("Output"=w263:dbl)
              }
            }
            n210 = flat-sequence {
              tunnel: w248 -> [w262]
              tunnel: [w259] -> w247
              frame #0 {
                # "Repetition 3"
                n211 = call "Math SubVI - Simple (PCR) (DBG OFF) (INLN).vi"("Input"=w262) -> ("Output"=w260:dbl)
                n212 = call "Math SubVI - Medium (PCR) (DBG OFF) (INLN).vi"("Input"=w260) -> ("Output"=w261:dbl)
                n213 = call "Math SubVI - Complex (PCR) (DBG OFF) (INLN).vi"("Input"=w261) -> ("Output"=w259:dbl)
              }
            }
            n214 = flat-sequence {
              tunnel: w247 -> [w258]
              tunnel: [w255] -> w246
              frame #0 {
                # "Repetition 4"
                n215 = call "Math SubVI - Simple (PCR) (DBG OFF) (INLN).vi"("Input"=w258) -> ("Output"=w256:dbl)
                n216 = call "Math SubVI - Medium (PCR) (DBG OFF) (INLN).vi"("Input"=w256) -> ("Output"=w257:dbl)
                n217 = call "Math SubVI - Complex (PCR) (DBG OFF) (INLN).vi"("Input"=w257) -> ("Output"=w255:dbl)
              }
            }
            n218 = flat-sequence {
              tunnel: w246 -> [w254]
              tunnel: [w251] -> w245
              frame #0 {
                # "Repetition 5"
                n219 = call "Math SubVI - Simple (PCR) (DBG OFF) (INLN).vi"("Input"=w254) -> ("Output"=w252:dbl)
                n220 = call "Math SubVI - Medium (PCR) (DBG OFF) (INLN).vi"("Input"=w252) -> ("Output"=w253:dbl)
                n221 = call "Math SubVI - Complex (PCR) (DBG OFF) (INLN).vi"("Input"=w253) -> ("Output"=w251:dbl)
              }
            }
          }
        }
        n222 = local read "Stop VI?"() -> (w218:bool)
      }
      n223 = for "Loop 6" {
        N: w18 -> [_]
        tunnel: [w160] -> w24 mode=indexing
        tunnel: [w161] -> w23
        i -> [w161]
        stop <- w162 stop-if-true
        n224 = Random Number (0-1)() -> (number: 0 to 1=w159:dbl)
        n225 = disable-structure shown="Enabled" {
          disable-tunnel: w159 -> [w168 w194]
          disable-tunnel: [w167 w189] -> w160
          frame Enabled {
            # "Case 1: Subroutines"
            n226 = flat-sequence {
              tunnel: w168 -> [w188]
              tunnel: [w185] -> w163
              frame #0 {
                # "Repetition 1"
                n227 = call "Math SubVI - Simple (PCR) (DBG OFF) (SBRTN).vi"("Input"=w188) -> ("Output"=w186:dbl)
                n228 = call "Math SubVI - Medium (PCR) (DBG OFF) (SBRTN).vi"("Input"=w186) -> ("Output"=w187:dbl)
                n229 = call "Math SubVI - Complex (PCR) (DBG OFF) (SBRTN).vi"("Input"=w187) -> ("Output"=w185:dbl)
              }
            }
            n230 = flat-sequence {
              tunnel: w163 -> [w184]
              tunnel: [w181] -> w166
              frame #0 {
                # "Repetition 2"
                n231 = call "Math SubVI - Simple (PCR) (DBG OFF) (SBRTN).vi"("Input"=w184) -> ("Output"=w182:dbl)
                n232 = call "Math SubVI - Medium (PCR) (DBG OFF) (SBRTN).vi"("Input"=w182) -> ("Output"=w183:dbl)
                n233 = call "Math SubVI - Complex (PCR) (DBG OFF) (SBRTN).vi"("Input"=w183) -> ("Output"=w181:dbl)
              }
            }
            n234 = flat-sequence {
              tunnel: w166 -> [w180]
              tunnel: [w177] -> w165
              frame #0 {
                # "Repetition 3"
                n235 = call "Math SubVI - Simple (PCR) (DBG OFF) (SBRTN).vi"("Input"=w180) -> ("Output"=w178:dbl)
                n236 = call "Math SubVI - Medium (PCR) (DBG OFF) (SBRTN).vi"("Input"=w178) -> ("Output"=w179:dbl)
                n237 = call "Math SubVI - Complex (PCR) (DBG OFF) (SBRTN).vi"("Input"=w179) -> ("Output"=w177:dbl)
              }
            }
            n238 = flat-sequence {
              tunnel: w165 -> [w176]
              tunnel: [w173] -> w164
              frame #0 {
                # "Repetition 4"
                n239 = call "Math SubVI - Simple (PCR) (DBG OFF) (SBRTN).vi"("Input"=w176) -> ("Output"=w174:dbl)
                n240 = call "Math SubVI - Medium (PCR) (DBG OFF) (SBRTN).vi"("Input"=w174) -> ("Output"=w175:dbl)
                n241 = call "Math SubVI - Complex (PCR) (DBG OFF) (SBRTN).vi"("Input"=w175) -> ("Output"=w173:dbl)
              }
            }
            n242 = flat-sequence {
              tunnel: w164 -> [w172]
              tunnel: [w169] -> w167
              frame #0 {
                # "Repetition 5"
                n243 = call "Math SubVI - Simple (PCR) (DBG OFF) (SBRTN).vi"("Input"=w172) -> ("Output"=w170:dbl)
                n244 = call "Math SubVI - Medium (PCR) (DBG OFF) (SBRTN).vi"("Input"=w170) -> ("Output"=w171:dbl)
                n245 = call "Math SubVI - Complex (PCR) (DBG OFF) (SBRTN).vi"("Input"=w171) -> ("Output"=w169:dbl)
              }
            }
          }
          frame Disabled {
            # "Case 2: Inline VIs"
            n246 = flat-sequence {
              tunnel: w194 -> [w214]
              tunnel: [w211] -> w193
              frame #0 {
                # "Repetition 1"
                n247 = call "Math SubVI - Simple (PCR) (DBG OFF) (INLN).vi"("Input"=w214) -> ("Output"=w212:dbl)
                n248 = call "Math SubVI - Medium (PCR) (DBG OFF) (INLN).vi"("Input"=w212) -> ("Output"=w213:dbl)
                n249 = call "Math SubVI - Complex (PCR) (DBG OFF) (INLN).vi"("Input"=w213) -> ("Output"=w211:dbl)
              }
            }
            n250 = flat-sequence {
              tunnel: w193 -> [w210]
              tunnel: [w207] -> w192
              frame #0 {
                # "Repetition 2"
                n251 = call "Math SubVI - Simple (PCR) (DBG OFF) (INLN).vi"("Input"=w210) -> ("Output"=w208:dbl)
                n252 = call "Math SubVI - Medium (PCR) (DBG OFF) (INLN).vi"("Input"=w208) -> ("Output"=w209:dbl)
                n253 = call "Math SubVI - Complex (PCR) (DBG OFF) (INLN).vi"("Input"=w209) -> ("Output"=w207:dbl)
              }
            }
            n254 = flat-sequence {
              tunnel: w192 -> [w206]
              tunnel: [w203] -> w191
              frame #0 {
                # "Repetition 3"
                n255 = call "Math SubVI - Simple (PCR) (DBG OFF) (INLN).vi"("Input"=w206) -> ("Output"=w204:dbl)
                n256 = call "Math SubVI - Medium (PCR) (DBG OFF) (INLN).vi"("Input"=w204) -> ("Output"=w205:dbl)
                n257 = call "Math SubVI - Complex (PCR) (DBG OFF) (INLN).vi"("Input"=w205) -> ("Output"=w203:dbl)
              }
            }
            n258 = flat-sequence {
              tunnel: w191 -> [w202]
              tunnel: [w199] -> w190
              frame #0 {
                # "Repetition 4"
                n259 = call "Math SubVI - Simple (PCR) (DBG OFF) (INLN).vi"("Input"=w202) -> ("Output"=w200:dbl)
                n260 = call "Math SubVI - Medium (PCR) (DBG OFF) (INLN).vi"("Input"=w200) -> ("Output"=w201:dbl)
                n261 = call "Math SubVI - Complex (PCR) (DBG OFF) (INLN).vi"("Input"=w201) -> ("Output"=w199:dbl)
              }
            }
            n262 = flat-sequence {
              tunnel: w190 -> [w198]
              tunnel: [w195] -> w189
              frame #0 {
                # "Repetition 5"
                n263 = call "Math SubVI - Simple (PCR) (DBG OFF) (INLN).vi"("Input"=w198) -> ("Output"=w196:dbl)
                n264 = call "Math SubVI - Medium (PCR) (DBG OFF) (INLN).vi"("Input"=w196) -> ("Output"=w197:dbl)
                n265 = call "Math SubVI - Complex (PCR) (DBG OFF) (INLN).vi"("Input"=w197) -> ("Output"=w195:dbl)
              }
            }
          }
        }
        n266 = local read "Stop VI?"() -> (w162:bool)
      }
      n267 = for "Loop 7" {
        N: w18 -> [_]
        tunnel: [w104] -> w22 mode=indexing
        tunnel: [w105] -> w21
        i -> [w105]
        stop <- w106 stop-if-true
        n268 = Random Number (0-1)() -> (number: 0 to 1=w103:dbl)
        n269 = disable-structure shown="Enabled" {
          disable-tunnel: w103 -> [w112 w138]
          disable-tunnel: [w111 w133] -> w104
          frame Enabled {
            # "Case 1: Subroutines"
            n270 = flat-sequence {
              tunnel: w112 -> [w132]
              tunnel: [w129] -> w107
              frame #0 {
                # "Repetition 1"
                n271 = call "Math SubVI - Simple (PCR) (DBG OFF) (SBRTN).vi"("Input"=w132) -> ("Output"=w130:dbl)
                n272 = call "Math SubVI - Medium (PCR) (DBG OFF) (SBRTN).vi"("Input"=w130) -> ("Output"=w131:dbl)
                n273 = call "Math SubVI - Complex (PCR) (DBG OFF) (SBRTN).vi"("Input"=w131) -> ("Output"=w129:dbl)
              }
            }
            n274 = flat-sequence {
              tunnel: w107 -> [w128]
              tunnel: [w125] -> w110
              frame #0 {
                # "Repetition 2"
                n275 = call "Math SubVI - Simple (PCR) (DBG OFF) (SBRTN).vi"("Input"=w128) -> ("Output"=w126:dbl)
                n276 = call "Math SubVI - Medium (PCR) (DBG OFF) (SBRTN).vi"("Input"=w126) -> ("Output"=w127:dbl)
                n277 = call "Math SubVI - Complex (PCR) (DBG OFF) (SBRTN).vi"("Input"=w127) -> ("Output"=w125:dbl)
              }
            }
            n278 = flat-sequence {
              tunnel: w110 -> [w124]
              tunnel: [w121] -> w109
              frame #0 {
                # "Repetition 3"
                n279 = call "Math SubVI - Simple (PCR) (DBG OFF) (SBRTN).vi"("Input"=w124) -> ("Output"=w122:dbl)
                n280 = call "Math SubVI - Medium (PCR) (DBG OFF) (SBRTN).vi"("Input"=w122) -> ("Output"=w123:dbl)
                n281 = call "Math SubVI - Complex (PCR) (DBG OFF) (SBRTN).vi"("Input"=w123) -> ("Output"=w121:dbl)
              }
            }
            n282 = flat-sequence {
              tunnel: w109 -> [w120]
              tunnel: [w117] -> w108
              frame #0 {
                # "Repetition 4"
                n283 = call "Math SubVI - Simple (PCR) (DBG OFF) (SBRTN).vi"("Input"=w120) -> ("Output"=w118:dbl)
                n284 = call "Math SubVI - Medium (PCR) (DBG OFF) (SBRTN).vi"("Input"=w118) -> ("Output"=w119:dbl)
                n285 = call "Math SubVI - Complex (PCR) (DBG OFF) (SBRTN).vi"("Input"=w119) -> ("Output"=w117:dbl)
              }
            }
            n286 = flat-sequence {
              tunnel: w108 -> [w116]
              tunnel: [w113] -> w111
              frame #0 {
                # "Repetition 5"
                n287 = call "Math SubVI - Simple (PCR) (DBG OFF) (SBRTN).vi"("Input"=w116) -> ("Output"=w114:dbl)
                n288 = call "Math SubVI - Medium (PCR) (DBG OFF) (SBRTN).vi"("Input"=w114) -> ("Output"=w115:dbl)
                n289 = call "Math SubVI - Complex (PCR) (DBG OFF) (SBRTN).vi"("Input"=w115) -> ("Output"=w113:dbl)
              }
            }
          }
          frame Disabled {
            # "Case 2: Inline VIs"
            n290 = flat-sequence {
              tunnel: w138 -> [w158]
              tunnel: [w155] -> w137
              frame #0 {
                # "Repetition 1"
                n291 = call "Math SubVI - Simple (PCR) (DBG OFF) (INLN).vi"("Input"=w158) -> ("Output"=w156:dbl)
                n292 = call "Math SubVI - Medium (PCR) (DBG OFF) (INLN).vi"("Input"=w156) -> ("Output"=w157:dbl)
                n293 = call "Math SubVI - Complex (PCR) (DBG OFF) (INLN).vi"("Input"=w157) -> ("Output"=w155:dbl)
              }
            }
            n294 = flat-sequence {
              tunnel: w137 -> [w154]
              tunnel: [w151] -> w136
              frame #0 {
                # "Repetition 2"
                n295 = call "Math SubVI - Simple (PCR) (DBG OFF) (INLN).vi"("Input"=w154) -> ("Output"=w152:dbl)
                n296 = call "Math SubVI - Medium (PCR) (DBG OFF) (INLN).vi"("Input"=w152) -> ("Output"=w153:dbl)
                n297 = call "Math SubVI - Complex (PCR) (DBG OFF) (INLN).vi"("Input"=w153) -> ("Output"=w151:dbl)
              }
            }
            n298 = flat-sequence {
              tunnel: w136 -> [w150]
              tunnel: [w147] -> w135
              frame #0 {
                # "Repetition 3"
                n299 = call "Math SubVI - Simple (PCR) (DBG OFF) (INLN).vi"("Input"=w150) -> ("Output"=w148:dbl)
                n300 = call "Math SubVI - Medium (PCR) (DBG OFF) (INLN).vi"("Input"=w148) -> ("Output"=w149:dbl)
                n301 = call "Math SubVI - Complex (PCR) (DBG OFF) (INLN).vi"("Input"=w149) -> ("Output"=w147:dbl)
              }
            }
            n302 = flat-sequence {
              tunnel: w135 -> [w146]
              tunnel: [w143] -> w134
              frame #0 {
                # "Repetition 4"
                n303 = call "Math SubVI - Simple (PCR) (DBG OFF) (INLN).vi"("Input"=w146) -> ("Output"=w144:dbl)
                n304 = call "Math SubVI - Medium (PCR) (DBG OFF) (INLN).vi"("Input"=w144) -> ("Output"=w145:dbl)
                n305 = call "Math SubVI - Complex (PCR) (DBG OFF) (INLN).vi"("Input"=w145) -> ("Output"=w143:dbl)
              }
            }
            n306 = flat-sequence {
              tunnel: w134 -> [w142]
              tunnel: [w139] -> w133
              frame #0 {
                # "Repetition 5"
                n307 = call "Math SubVI - Simple (PCR) (DBG OFF) (INLN).vi"("Input"=w142) -> ("Output"=w140:dbl)
                n308 = call "Math SubVI - Medium (PCR) (DBG OFF) (INLN).vi"("Input"=w140) -> ("Output"=w141:dbl)
                n309 = call "Math SubVI - Complex (PCR) (DBG OFF) (INLN).vi"("Input"=w141) -> ("Output"=w139:dbl)
              }
            }
          }
        }
        n310 = local read "Stop VI?"() -> (w106:bool)
      }
      n311 = for "Loop 8" {
        N: w18 -> [_]
        tunnel: [w48] -> w19 mode=indexing
        tunnel: [w49] -> w20
        i -> [w49]
        stop <- w50 stop-if-true
        n312 = Random Number (0-1)() -> (number: 0 to 1=w47:dbl)
        n313 = disable-structure shown="Enabled" {
          disable-tunnel: w47 -> [w56 w82]
          disable-tunnel: [w55 w77] -> w48
          frame Enabled {
            # "Case 1: Subroutines"
            n314 = flat-sequence {
              tunnel: w56 -> [w76]
              tunnel: [w73] -> w51
              frame #0 {
                # "Repetition 1"
                n315 = call "Math SubVI - Simple (PCR) (DBG OFF) (SBRTN).vi"("Input"=w76) -> ("Output"=w74:dbl)
                n316 = call "Math SubVI - Medium (PCR) (DBG OFF) (SBRTN).vi"("Input"=w74) -> ("Output"=w75:dbl)
                n317 = call "Math SubVI - Complex (PCR) (DBG OFF) (SBRTN).vi"("Input"=w75) -> ("Output"=w73:dbl)
              }
            }
            n318 = flat-sequence {
              tunnel: w51 -> [w72]
              tunnel: [w69] -> w54
              frame #0 {
                # "Repetition 2"
                n319 = call "Math SubVI - Simple (PCR) (DBG OFF) (SBRTN).vi"("Input"=w72) -> ("Output"=w70:dbl)
                n320 = call "Math SubVI - Medium (PCR) (DBG OFF) (SBRTN).vi"("Input"=w70) -> ("Output"=w71:dbl)
                n321 = call "Math SubVI - Complex (PCR) (DBG OFF) (SBRTN).vi"("Input"=w71) -> ("Output"=w69:dbl)
              }
            }
            n322 = flat-sequence {
              tunnel: w54 -> [w68]
              tunnel: [w65] -> w53
              frame #0 {
                # "Repetition 3"
                n323 = call "Math SubVI - Simple (PCR) (DBG OFF) (SBRTN).vi"("Input"=w68) -> ("Output"=w66:dbl)
                n324 = call "Math SubVI - Medium (PCR) (DBG OFF) (SBRTN).vi"("Input"=w66) -> ("Output"=w67:dbl)
                n325 = call "Math SubVI - Complex (PCR) (DBG OFF) (SBRTN).vi"("Input"=w67) -> ("Output"=w65:dbl)
              }
            }
            n326 = flat-sequence {
              tunnel: w53 -> [w64]
              tunnel: [w61] -> w52
              frame #0 {
                # "Repetition 4"
                n327 = call "Math SubVI - Simple (PCR) (DBG OFF) (SBRTN).vi"("Input"=w64) -> ("Output"=w62:dbl)
                n328 = call "Math SubVI - Medium (PCR) (DBG OFF) (SBRTN).vi"("Input"=w62) -> ("Output"=w63:dbl)
                n329 = call "Math SubVI - Complex (PCR) (DBG OFF) (SBRTN).vi"("Input"=w63) -> ("Output"=w61:dbl)
              }
            }
            n330 = flat-sequence {
              tunnel: w52 -> [w60]
              tunnel: [w57] -> w55
              frame #0 {
                # "Repetition 5"
                n331 = call "Math SubVI - Simple (PCR) (DBG OFF) (SBRTN).vi"("Input"=w60) -> ("Output"=w58:dbl)
                n332 = call "Math SubVI - Medium (PCR) (DBG OFF) (SBRTN).vi"("Input"=w58) -> ("Output"=w59:dbl)
                n333 = call "Math SubVI - Complex (PCR) (DBG OFF) (SBRTN).vi"("Input"=w59) -> ("Output"=w57:dbl)
              }
            }
          }
          frame Disabled {
            # "Case 2: Inline VIs"
            n334 = flat-sequence {
              tunnel: w82 -> [w102]
              tunnel: [w99] -> w81
              frame #0 {
                # "Repetition 1"
                n335 = call "Math SubVI - Simple (PCR) (DBG OFF) (INLN).vi"("Input"=w102) -> ("Output"=w100:dbl)
                n336 = call "Math SubVI - Medium (PCR) (DBG OFF) (INLN).vi"("Input"=w100) -> ("Output"=w101:dbl)
                n337 = call "Math SubVI - Complex (PCR) (DBG OFF) (INLN).vi"("Input"=w101) -> ("Output"=w99:dbl)
              }
            }
            n338 = flat-sequence {
              tunnel: w81 -> [w98]
              tunnel: [w95] -> w80
              frame #0 {
                # "Repetition 2"
                n339 = call "Math SubVI - Simple (PCR) (DBG OFF) (INLN).vi"("Input"=w98) -> ("Output"=w96:dbl)
                n340 = call "Math SubVI - Medium (PCR) (DBG OFF) (INLN).vi"("Input"=w96) -> ("Output"=w97:dbl)
                n341 = call "Math SubVI - Complex (PCR) (DBG OFF) (INLN).vi"("Input"=w97) -> ("Output"=w95:dbl)
              }
            }
            n342 = flat-sequence {
              tunnel: w80 -> [w94]
              tunnel: [w91] -> w79
              frame #0 {
                # "Repetition 3"
                n343 = call "Math SubVI - Simple (PCR) (DBG OFF) (INLN).vi"("Input"=w94) -> ("Output"=w92:dbl)
                n344 = call "Math SubVI - Medium (PCR) (DBG OFF) (INLN).vi"("Input"=w92) -> ("Output"=w93:dbl)
                n345 = call "Math SubVI - Complex (PCR) (DBG OFF) (INLN).vi"("Input"=w93) -> ("Output"=w91:dbl)
              }
            }
            n346 = flat-sequence {
              tunnel: w79 -> [w90]
              tunnel: [w87] -> w78
              frame #0 {
                # "Repetition 4"
                n347 = call "Math SubVI - Simple (PCR) (DBG OFF) (INLN).vi"("Input"=w90) -> ("Output"=w88:dbl)
                n348 = call "Math SubVI - Medium (PCR) (DBG OFF) (INLN).vi"("Input"=w88) -> ("Output"=w89:dbl)
                n349 = call "Math SubVI - Complex (PCR) (DBG OFF) (INLN).vi"("Input"=w89) -> ("Output"=w87:dbl)
              }
            }
            n350 = flat-sequence {
              tunnel: w78 -> [w86]
              tunnel: [w83] -> w77
              frame #0 {
                # "Repetition 5"
                n351 = call "Math SubVI - Simple (PCR) (DBG OFF) (INLN).vi"("Input"=w86) -> ("Output"=w84:dbl)
                n352 = call "Math SubVI - Medium (PCR) (DBG OFF) (INLN).vi"("Input"=w84) -> ("Output"=w85:dbl)
                n353 = call "Math SubVI - Complex (PCR) (DBG OFF) (INLN).vi"("Input"=w85) -> ("Output"=w83:dbl)
              }
            }
          }
        }
        n354 = local read "Stop VI?"() -> (w50:bool)
      }
      n355 = call <vilib>:"High Resolution Polling Wait.vi"("seconds to wait"=w44) -> ("error out"=w43:errorcluster)  [unwired: 10 in]
      n356 = flat-sequence {
        tunnel: w43 -> [w45]
        frame #0 {
          n357 = call <vilib>:"Clear Errors.vi"("error in (no error)"=w45) -> ()  [unwired: 5 in, 2 out]
          "Stop VI?" <- TRUE
        }
      }
      n358 = Increment(x=w25) -> (x+1=w36:i32)
      n359 = Increment(x=w23) -> (x+1=w33:i32)
      n360 = Increment(x=w21) -> (x+1=w34:i32)
      n361 = Increment(x=w20) -> (x+1=w35:i32)
      n362 = Increment(x=w41) -> (x+1=w40:i32)
      n363 = Increment(x=w31) -> (x+1=w39:i32)
      n364 = Increment(x=w29) -> (x+1=w38:i32)
      n365 = Increment(x=w27) -> (x+1=w37:i32)
    }
    frame #2 {
      n366 = Build Array(w515, w514, w510, w509, w503, w502, w501, w500) -> (w499:i32[])
      n367 = for {
        tunnel: w499 -> [w521] mode=indexing
        tunnel: [w520] -> w498 mode=indexing
        n368 = Number To Decimal String(number=w521) -> (decimal integer string=w520:string)  [unwired: 1 in]
      }
      n369 = To Double Precision Float(number=w499) -> (double precision float=w508:dbl[])
      n370 = call-poly <vilib>:"Mean.vi"("X"=w508) -> ("mean"=w513:dbl)  [unwired: 1 out]
      "Avg. No. Of Iterations Executed - All Loops" <- w513
      n371 = disable-structure shown="Enabled" {
        disable-tunnel: w513 -> [w519 _]
        frame Disabled {
          n372 = call "Copy Result To Clipboard.vi"("No. Of Decimal Places (6)"=u32 1, "Input"=w519) -> ()
        }
        frame Enabled {
        }
      }
      n373 = call-poly <vilib>:"1D String Array to Delimited String.vi"("delimiter"="\r\n", "string array"=w498) -> ("delimited string"=w495:string)  [unwired: 9 in]
      "No. Of Iterations As Block Of Text (easy to copy into Excel)" <- w495
      n374 = invoke class="Application" method="Clipboard.Write"("Param 0"=w495) -> (error out=w496:errorcluster)  [unwired: 3 in, 3 out]
      n375 = call <vilib>:"Clear Errors.vi"("error in (no error)"=w496) -> ()  [unwired: 5 in, 2 out]
      "No. Of Iterations Executed - Loop 1" <- w515
      "Output - Loop 1" <- w517
      "No. Of Iterations Executed - Loop 2" <- w514
      "Output - Loop 2" <- w516
      "No. Of Iterations Executed - Loop 3" <- w510
      "Output - Loop 3" <- w512
      "No. Of Iterations Executed - Loop 4" <- w509
      "Output - Loop 4" <- w511
      "No. Of Iterations Executed - Loop 5" <- w503
      "Output - Loop 5" <- w507
      "No. Of Iterations Executed - Loop 6" <- w502
      "Output - Loop 6" <- w506
      "No. Of Iterations Executed - Loop 7" <- w501
      "Output - Loop 7" <- w505
      "No. Of Iterations Executed - Loop 8" <- w500
      "Output - Loop 8" <- w504
    }
  }
